vi "write_controller_file.vi"(6 "5V reg":cluster{u16, u16}, 7 "3.3V reg":cluster{u16, u16}, 9 "BUS":cluster{u16, u16, u16}, 10 "minutes":dbl, 11 "controller file":path) -> ()   [LabVIEW 2019]
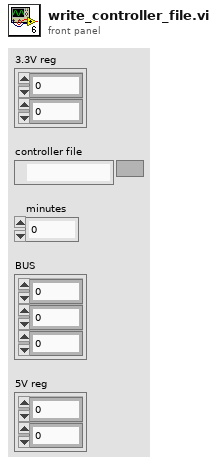
[diagram p1: front panel]
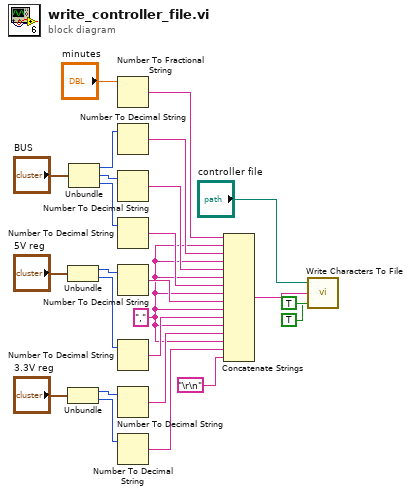
[diagram p0: block diagram]
diagram:
  w1 = "," ("string")
  n1 = Unbundle("5V reg") -> (w23:u16, w10:u16)
  n2 = Unbundle("3.3V reg") -> (w9:u16, w8:u16)
  n3 = Unbundle("BUS") -> (w15:u16, w16:u16, w17:u16)
  n4 = Number To Fractional String(number="minutes") -> (F-format string=w18:string)  [unwired: 3 in]
  n5 = Number To Decimal String(number=w15) -> (decimal integer string=w19:string)  [unwired: 1 in]
  n6 = Number To Decimal String(number=w16) -> (decimal integer string=w20:string)  [unwired: 1 in]
  n7 = Number To Decimal String(number=w17) -> (decimal integer string=w2:string)  [unwired: 1 in]
  n8 = Number To Decimal String(number=w23) -> (decimal integer string=w3:string)  [unwired: 1 in]
  n9 = Number To Decimal String(number=w10) -> (decimal integer string=w4:string)  [unwired: 1 in]
  n10 = Number To Decimal String(number=w9) -> (decimal integer string=w5:string)  [unwired: 1 in]
  n11 = Number To Decimal String(number=w8) -> (decimal integer string=w6:string)  [unwired: 1 in]
  n12 = Concatenate Strings(w18, w1, w19, w1, w20, w1, w2, w1, w3, w1, w4, w1, w5, w1, w6, "\r\n") -> (w24:string)
  n13 = call <vilib>:"Write Characters To File.vi"("convert eol? (no:F)"=TRUE, "append to file? (new file:F)"=TRUE, "character string"=w24, "file path (dialog if empty)"="controller file") -> ()  [unwired: 1 in, 1 out]
